vi "KM101_MoveAbsoluteStep.vi"(8 "bWait":bool, 9 "AbsSteps":i32, 10 "Channel":i32, 11 "reference in":refnum<k7>) -> (2 "reference out":refnum<k7>)   [LabVIEW 2018, in "KIM101lib.lvlib"]
uses:
  KIM101lib.lvlib
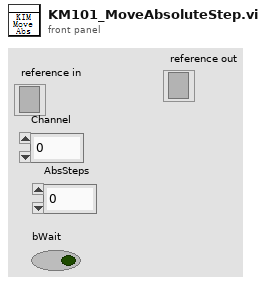
[diagram p1: front panel]
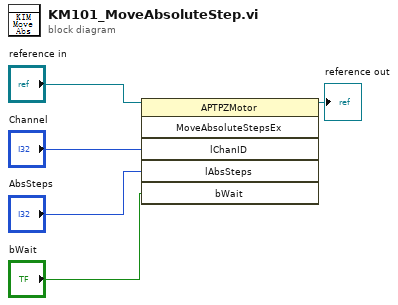
[diagram p0: block diagram]
diagram:
  n1 = invoke class="APTPZMotor" method="MoveAbsoluteStepsEx"(reference="reference in", "lChanID"="Channel", "lAbsSteps"="AbsSteps", "bWait"="bWait") -> (reference out=→"reference out":refnum<k7>)  [unwired: 2 in, 5 out]
